vi "Write to Log File (Waveform).vi"(6 "Waveform Data":waveform(dbl)[](array[waveform]), 8 "error in (no error)":errorcluster, 9 "Channel Names in":string[](array[string]), 10 "Group Names in":string[](array[string]), 11 "Log File in":refnum<class "Log File.lvclass">) -> (0 "error out":errorcluster, 3 "Log File out":refnum<class "Log File.lvclass">)   [LabVIEW 2015, in "Waveform Data Logger Engine.lvlib" / "Log File.lvclass"]
uses:
  Log File.lvclass
  Log File.lvclass/Log File.ctl
  TDMS Log File/TDMS Log File.lvclass
  Text Log File/Text Log File.lvclass
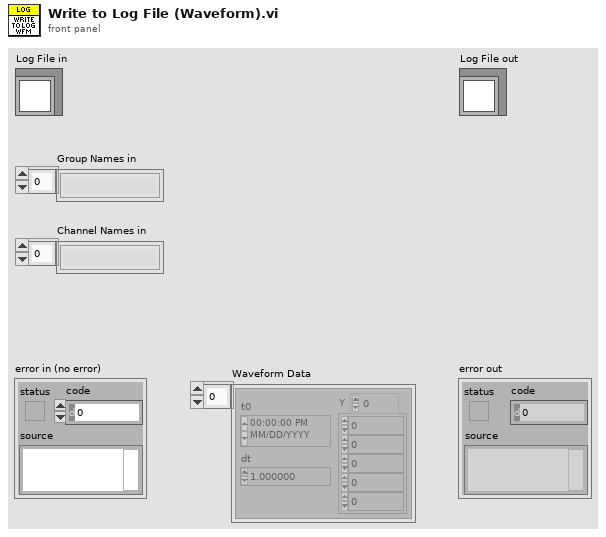
[diagram p1: front panel]
types:
  T1 = typedef "Waveform Data Logger Engine.lvlib/Log File.lvclass/Log File Type.ctl" = enum16{"Default", "TDMS", "Text"}
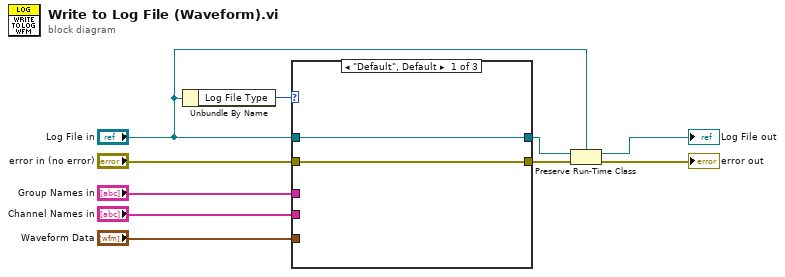
[diagram p0: block diagram]
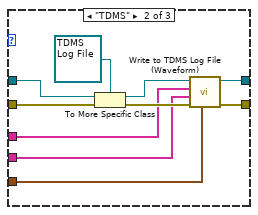
[diagram p2: hidden frame]
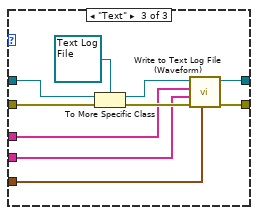
[diagram p3: hidden frame]
diagram:
  n1 = Unbundle By Name("Log File in") -> ("Log File Type"=w10:T1)
  n2 = case shown="\"Default\", Default" w10 {
    tunnel: "error in (no error)" -> [w12 w22 w31]
    tunnel: [w12 w17 w32] -> w5
    tunnel: "Log File in" -> [w11 w21 w29]
    tunnel: [w11 w16 w26] -> w4
    tunnel: "Waveform Data" -> [_ w13 w23]
    tunnel: "Group Names in" -> [_ w15 w24]
    tunnel: "Channel Names in" -> [_ w14 w25]
    frame "Default", Default {
    }
    frame "TDMS" {
      n3 = To More Specific Class(target class=refnum<class "TDMS Log File.lvclass"> refnum ("TDMS Log File.lvclass"), reference=w21, error in=w22) -> (specific class reference=w19:refnum<class "TDMS Log File.lvclass">, error out=w18:errorcluster)
      n4 = call "Write to TDMS Log File (Waveform).vi"("Waveform Data"=w13, "error in (no error)"=w18, "Channel Names in"=w14, "Group Names in"=w15, "TDMS Log File in"=w19) -> ("error out"=w17:errorcluster, "TDMS Log File out"=w16:refnum<class "TDMS Log File.lvclass">)  [unwired: 5 in]
    }
    frame "Text" {
      n5 = To More Specific Class(target class=refnum<class "Text Log File.lvclass"> refnum ("Text Log File.lvclass"), reference=w29, error in=w31) -> (specific class reference=w27:refnum<class "Text Log File.lvclass">, error out=w30:errorcluster)
      n6 = call "Write to Text Log File (Waveform).vi"("Waveform Data"=w23, "error in (no error)"=w30, "Channel Names in"=w25, "Group Names in"=w24, "Text Log File in"=w27) -> ("error out"=w32:errorcluster, "Text Log File out"=w26:refnum<class "Text Log File.lvclass">)  [unwired: 5 in]
    }
  }
  n7 = Preserve Run-Time Class(object in=w4, error in=w5, 2:"Log File in") -> (object out=→"Log File out":refnum<class "Log File.lvclass">, error out=→"error out":errorcluster)
